vi "pilot&controller.vi"() -> (3 "data":string caption="데이터")   [LabVIEW 2014]
uses:
  <vilib>/FTP/NI_FTP.lvlib
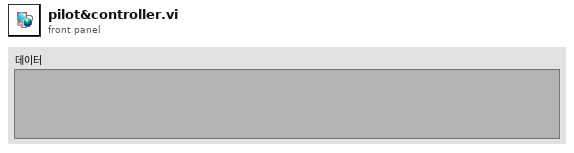
[diagram p1: front panel]
types:
  T1 = typedef "NI_FTP.lvlib/FTP Session.ctl" = refnum<k5>
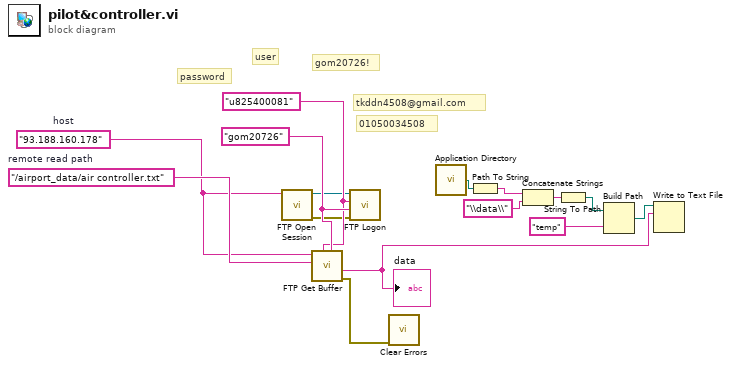
[diagram p0: block diagram]
diagram:
  w13 = "gom20726"
  w12 = "u825400081"
  w15 = "/airport_data/air controller.txt"  # remote read path
  w14 = "93.188.160.178"  # host
  # "gom20726!"
  # "01050034508"
  # "tkddn4508@gmail.com"
  # "user"
  # "password"
  n1 = call <vilib>:"FTP Open Session.vi"("address"=w14) -> ("error out"=w11:errorcluster, "ftp session"=w10:T1)  [unwired: 7 in, 2 out]
  n2 = call <vilib>:"FTP Get Buffer.vi"("password"=w13, "user"=w12, "remote path"=w15, "host"=w14) -> ("error out"=w1:errorcluster, "data"=w3:string)  [unwired: 5 in, 1 out]
  "data" <- w3
  n3 = call <vilib>:"FTP Logon.vi"("error in (no error)"=w11, "password"=w13, "user"=w12, "ftp session"=w10) -> ()  [unwired: 4 in, 4 out]
  n4 = call <vilib>:"Clear Errors.vi"("error in (no error)"=w1) -> ()  [unwired: 5 in, 2 out]
  n5 = call <vilib>:"Application Directory.vi"() -> ("Application Directory"=w8:path)
  n6 = Path To String(path=w8) -> (string=w7:string)
  n7 = Concatenate Strings(w7, "\\data\\" ("문자열")) -> (w6:string)
  n8 = String To Path(string=w6) -> (path=w4:path)
  n9 = Build Path(base path=w4, name or relative path="temp" ("이름 또는 상대 경로")) -> (appended path=w5:path)
  n10 = Write to Text File(file (use dialog)=w5, text=w3) -> ()  [unwired: 2 in, 3 out]
